vi "SetWaveforms.vi"(8 "error in (no error)":errorcluster, 10 "Waveforms":waveform(dbl)[](array[waveform]), 11 "ArbitraryFunction in":refnum<class "ArbitraryFunction.lvclass">) -> (0 "error out":errorcluster, 3 "ArbitraryFunction out":refnum<class "ArbitraryFunction.lvclass">)   [LabVIEW 2018, in "Functions.lvlib" / "ArbitraryFunction.lvclass"]
uses:
  ArbitraryFunction.lvclass
  ArbitraryFunction.lvclass/ArbitraryFunction.ctl
  Accessors/Read Arbs.vi
  Accessors/Write Arbs.vi
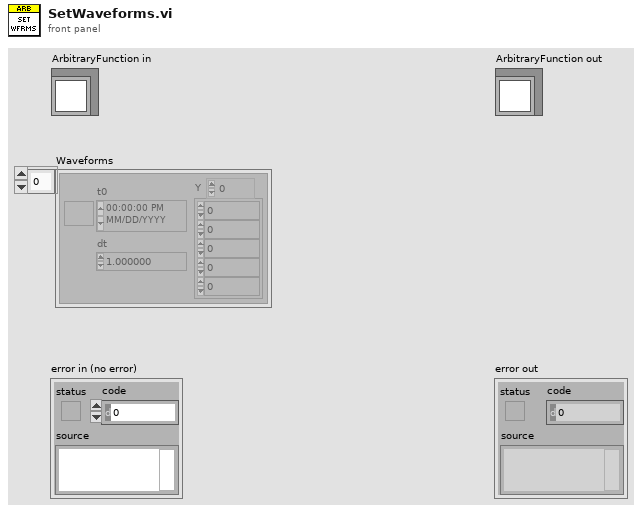
[diagram p1: front panel]
types:
  T1 = typedef "Functions.lvlib/ArbitraryFunction.lvclass/Arbitrary.ctl" = cluster{"Handle":string, "Size":i32, "Gain":dbl, "Offset":dbl, "Waveform":waveform(dbl)}
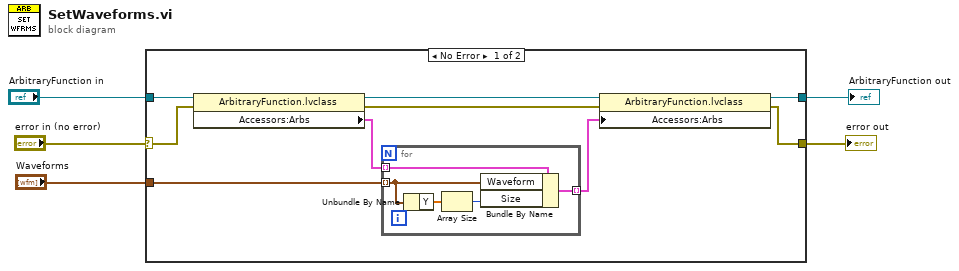
[diagram p0: block diagram]
diagram:
  n1 = case shown="No Error" "error in (no error)" {
    selector: "error in (no error)" -> [w11 w20]
    tunnel: "ArbitraryFunction in" -> [w14 w21]
    tunnel: "Waveforms" -> [w12 _]
    tunnel: [w7 w21] -> w2
    tunnel: [w6 w20] -> w1
    frame No Error {
      n2 = property class="ArbitraryFunction.lvclass"(reference=w14, error in=w11) -> (reference out=w10:refnum<class "ArbitraryFunction.lvclass">, error out=w8:errorcluster, "Accessors:Arbs"=w13:T1[])
      n3 = for {
        tunnel: w13 -> [w19] mode=indexing
        tunnel: w12 -> [w17] mode=indexing
        tunnel: [w18] -> w9 mode=indexing
        n4 = Unbundle By Name(w17) -> ("Y"=w15:dbl[])
        n5 = Array Size(array=w15) -> (size(s)=w16:i32)
        n6 = Bundle By Name(cluster=w19, "Waveform"=w17, "Size"=w16) -> (w18:T1)
      }
      n7 = property class="ArbitraryFunction.lvclass"(reference=w10, error in=w8, "Accessors:Arbs"=w9) -> (reference out=w7:refnum<class "ArbitraryFunction.lvclass">, error out=w6:errorcluster)
    }
    frame Error {
    }
  }
  "error out" <- w1
  "ArbitraryFunction out" <- w2
